vi "Write Transient temporarily.vi"(8 "error in (no error)":errorcluster, 10 "Transient Gains 2":T1, 11 "Data Analyser Report in":refnum<class "Data Analyser Report.lvclass">) -> (0 "error out":errorcluster, 3 "Data Analyser Report out":refnum<class "Data Analyser Report.lvclass">)   [LabVIEW 2016, in "Data Analyser Report.lvclass"]
uses:
  Data Analyser Report.lvclass
  C:/Users/w.figtree/Desktop/Work/4. Projects/3. In Progress Engineering Projects/EMA/src/core/Classes/Excel Interface/Excel Sheet/Excel Sheet.lvclass
  Excel Interface/Excel Sheet/Write to Cell - String.vi
  Excel Interface/Excel Sheet/Excel Sheet.lvclass
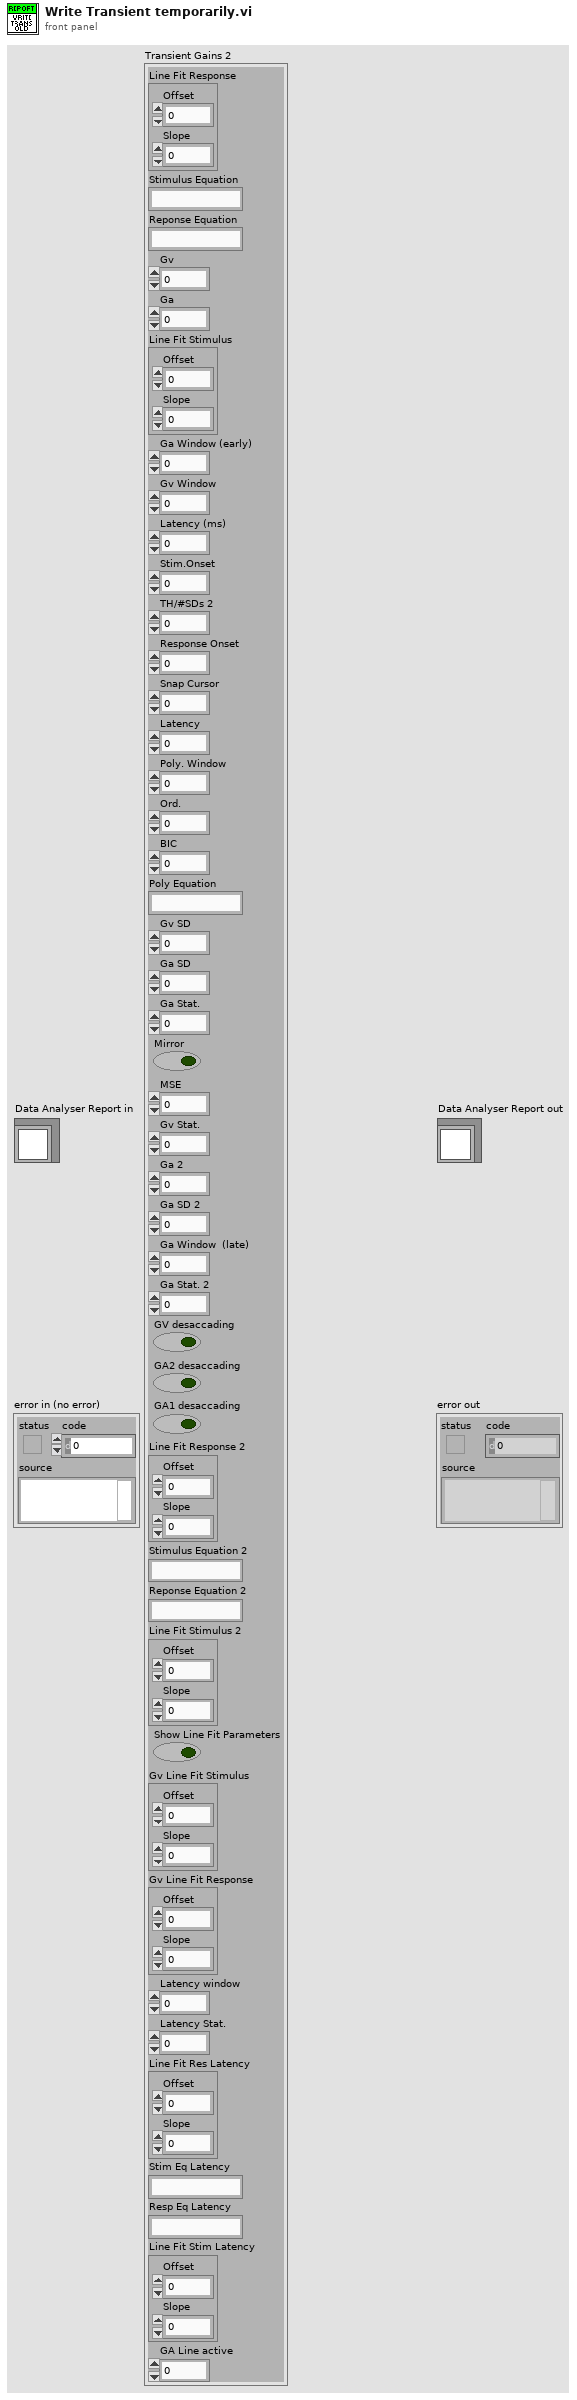
[diagram p1: front panel]
types:
  T1 = cluster{"Line Fit Response":cluster{"Offset":dbl, "Slope":dbl}, "Stimulus Equation":string, "Reponse Equation":string, "Gv":dbl, "Ga":dbl, "Line Fit Stimulus":cluster{"Offset":dbl, "Slope":dbl}, "Ga Window (early)":u16, "Gv Window":u16, "Latency (ms)":dbl, "Stim.Onset":dbl, "TH/#SDs 2":dbl, "Response Onset":dbl, "Snap Cursor":u16, "Latency":u16, "Poly. Window":u16, "Ord.":i32, "BIC":dbl, "Poly Equation":string, "Gv SD":dbl, "Ga SD":dbl, "Ga Stat.":u16, "Mirror":bool, "MSE":dbl, "Gv Stat.":u16, "Ga 2":dbl, "Ga SD 2":dbl, "Ga Window  (late)":u16, "Ga Stat. 2":u16, "GV desaccading":bool, "GA2 desaccading":bool, "GA1 desaccading":bool, "Line Fit Response 2":cluster{"Offset":dbl, "Slope":dbl}, "Stimulus Equation 2":string, "Reponse Equation 2":string, "Line Fit Stimulus 2":cluster{"Offset":dbl, "Slope":dbl}, "Show Line Fit Parameters ":bool, "Gv Line Fit Stimulus":cluster{"Offset":dbl, "Slope":dbl}, "Gv Line Fit Response":cluster{"Offset":dbl, "Slope":dbl}, "Latency window":u16, "Latency Stat.":u16, "Line Fit Res Latency":cluster{"Offset":dbl, "Slope":dbl}, "Stim Eq Latency":string, "Resp Eq Latency":string, "Line Fit Stim Latency":cluster{"Offset":dbl, "Slope":dbl}, "GA Line active":i32}
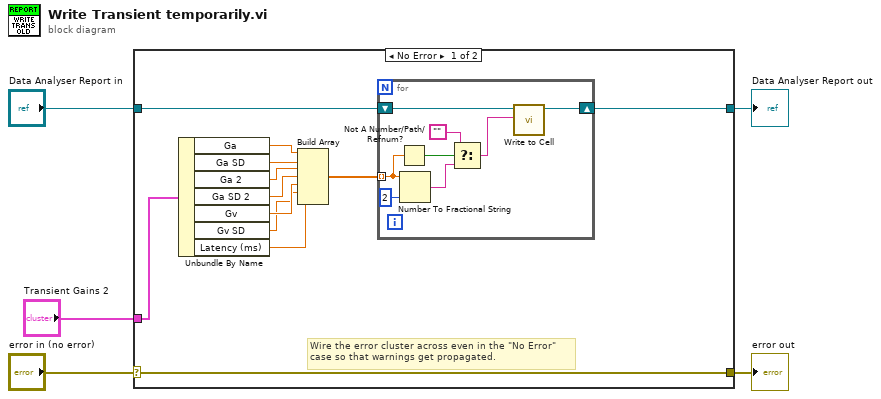
[diagram p0: block diagram]
diagram:
  n1 = case shown="No Error" "error in (no error)" {
    selector: "error in (no error)" -> [w17 w27]
    tunnel: [w17 w27] -> w4
    tunnel: [w15 w26] -> w2
    tunnel: "Data Analyser Report in" -> [w16 w26]
    tunnel: "Transient Gains 2" -> [w14 _]
    frame No Error {
      # "Wire the error cluster across even in the \"No Error\"\ncase so that warnings get propagated."
      n2 = Unbundle By Name(w14) -> ("Ga"=w12:dbl, "Ga SD"=w11:dbl, "Ga 2"=w13:dbl, "Ga SD 2"=w10:dbl, "Gv"=w9:dbl, "Gv SD"=w8:dbl, "Latency (ms)"=w7:dbl)
      n3 = Build Array(w12, w11, w13, w10, w9, w8, w7) -> (w6:dbl[])
      n4 = for {
        shift-right: [w24] -> w15
        shift-left: w16 -> [w25]
        tunnel: w6 -> [w22] mode=indexing
        n5 = Not A Number/Path/Refnum?(number/path/refnum=w22) -> (NaN/Path/Refnum?=w21:bool)
        n6 = Number To Fractional String(number=w22, precision (6)=i16 2) -> (F-format string=w20:string)  [unwired: 2 in]
        n7 = Select(t="", s=w21, f=w20) -> (s? t:f=w19:string)
        n8 = call-poly "Write to Cell.vi"("Value"=w19, "Excel Sheet in"=w25) -> ("Excel Sheet out"=w24:refnum<class "Data Analyser Report.lvclass">)  [unwired: 9 in]
      }
    }
    frame Error {
    }
  }
  "error out" <- w4
  "Data Analyser Report out" <- w2
